vi "test.vi"() -> ()   [LabVIEW 2010]
uses:
  <vilib>/vision/NI_Vision_Development_Module.lvlib
panel:
  out "data value":u8[](array[numeric])
  out "Data string":string
  out "LineWidth(Pixels)":i32
  out "Pixel Size (Bytes)":i32
  out "Pixel Pointer out":u64 format="%.0x"
  out "Image":T1(plugin-control)
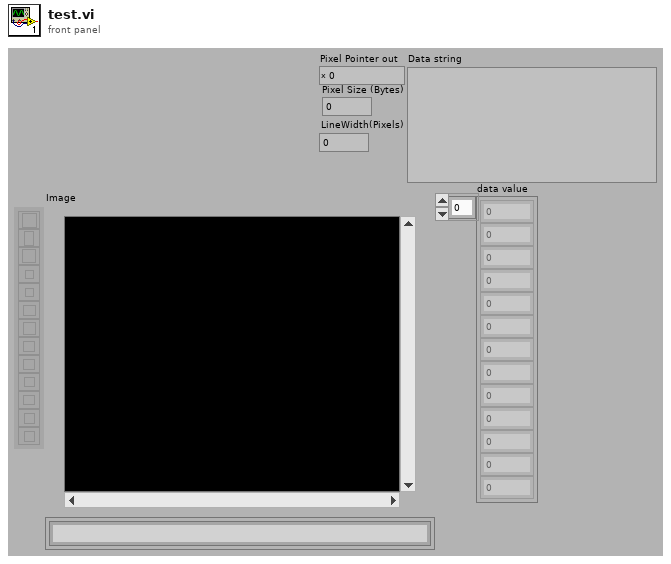
[diagram p1: front panel]
types:
  T1 = typedef "IMAQ Image.ctl" = refnum<image>
  T2 = enum32{"Map Pixel Pointer", "Unmap Pixel Pointer", "Get Pixels Infos"}
  T3 = typedef "Image Type" = u32
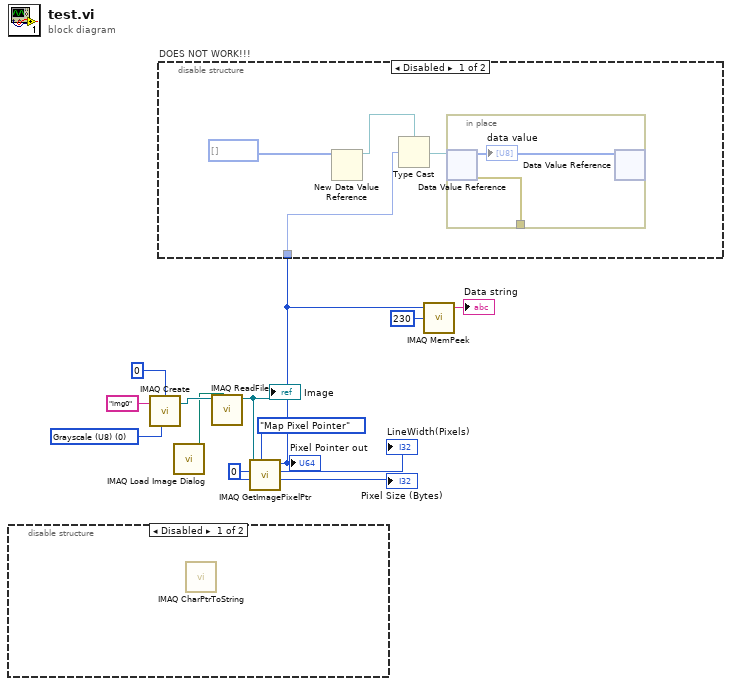
[diagram p0: block diagram]
diagram:
  w9 = 0 ("X Coordinate")
  w12 = T3 0 items=["Grayscale (U8)", "Grayscale (I16)", "Grayscale (SGL)", "Complex (CSG)", "RGB (U32)", "HSL (U32)", "RGB (U64)", "Grayscale (U16)"] ("Image Type")
  n1 = disable-structure shown="Disabled" {
    frame Disabled {
      n2 = call "IMAQ CharPtrToString"() -> ()  [unwired: 5 in, 2 out]
    }
    frame Enabled {
    }
  }
  n3 = call "IMAQ Create"("Border Size"=0, "Image Name"="img0", "Image Type"=w12) -> ("New Image"=w11:T1)  [unwired: 2 in, 1 out]
  n4 = call "IMAQ Load Image Dialog"() -> ("Path"=w10:path)  [unwired: 9 in, 2 out]
  n5 = call "IMAQ ReadFile"("File Path"=w10, "Image"=w11) -> ("Image Out"=w2:T1)  [unwired: 5 in, 4 out]
  "Image" <- w2
  n6 = call "IMAQ GetImagePixelPtr"("Function"=T2."Map Pixel Pointer", "Y Coordinate"=w9, "X Coordinate"=w9, "Image"=w2) -> ("Pixel Size (Bytes)"=→"Pixel Size (Bytes)":i32, "LineWidth(Pixels)"=→"LineWidth(Pixels)":i32, "Pixel Pointer out"=w1:u64)  [unwired: 2 in, 3 out]
  "Pixel Pointer out" <- w1
  n7 = disable-structure "DOES NOT WORK!!!" shown="Disabled" {
    disable-tunnel: w1 -> [w14 _]
    frame Disabled {
      n8 = New Data Value Reference(data value=u8[] []) -> (data value reference=w17:refnum<data-value>)  [unwired: 1 in, 1 out]
      n9 = Type Cast(type=w17, x=w14) -> (*(type *) &x=w16:refnum<data-value>)
      n10 = in-place {
        in-place-border: [w18] -> _
        n11 = in-place-dvr #1(w16) -> (w19:u8[], w18:errorcluster)
        "data value" <- w19
        n12 = in-place-dvr #1(w19) -> ()  [unwired: 2 out]
      }
    }
    frame Enabled {
    }
  }
  n13 = call "IMAQ MemPeek"("Bytes count"=230, "void*"=w1) -> ("Data string"=→"Data string":string)  [unwired: 2 in, 1 out]
